vi "_FPGA_Driver_V1.4DIO.vi"(10 "DO":u8) -> (2 "DI":u8)   [LabVIEW 2018]
uses:
  <vilib>/rvi/eio/common/nirviEmuTemplateMethod_errors.vi
  <vilib>/eio/EIONode/EIONode.xnode
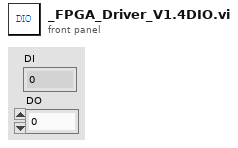
[diagram p1: front panel]
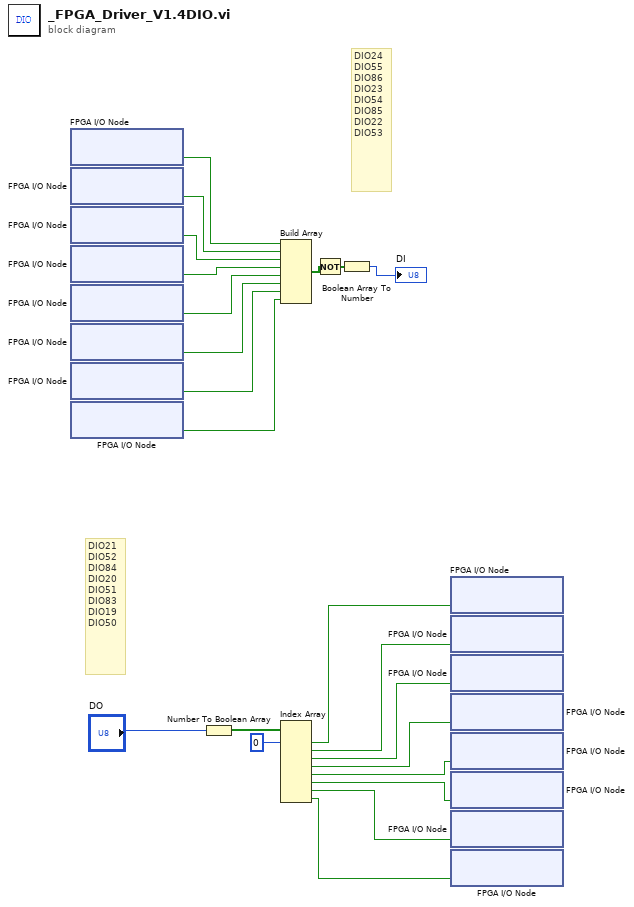
[diagram p0: block diagram]
diagram:
  # "DIO21\nDIO52\nDIO84\nDIO20\nDIO51\nDIO83\nDIO19\nDIO50"
  # "DIO24\nDIO55\nDIO86\nDIO23\nDIO54\nDIO85\nDIO22\nDIO53"
  n1 = xnode "FPGA I/O Node"() -> ("RMC/DIO24"=w22:bool)  [unwired: 1 in, 1 out]
  n2 = xnode "FPGA I/O Node"() -> ("RMC/DIO55"=w21:bool)  [unwired: 1 in, 1 out]
  n3 = xnode "FPGA I/O Node"() -> ("RMC/DIO86"=w20:bool)  [unwired: 1 in, 1 out]
  n4 = xnode "FPGA I/O Node"() -> ("RMC/DIO23"=w19:bool)  [unwired: 1 in, 1 out]
  n5 = xnode "FPGA I/O Node"() -> ("RMC/DIO54"=w18:bool)  [unwired: 1 in, 1 out]
  n6 = xnode "FPGA I/O Node"() -> ("RMC/DIO85"=w17:bool)  [unwired: 1 in, 1 out]
  n7 = xnode "FPGA I/O Node"() -> ("RMC/DIO22"=w16:bool)  [unwired: 1 in, 1 out]
  n8 = xnode "FPGA I/O Node"() -> ("RMC/DIO53"=w15:bool)  [unwired: 1 in, 1 out]
  n9 = Number To Boolean Array(number="DO") -> (Boolean array=w11:bool[])
  n10 = Build Array(w22, w21, w20, w19, w18, w17, w16, w15) -> (w14:bool[])
  n11 = Index Array(array=w11, index #1=0 ("index")) -> (element #1=w9:bool, element #2=w8:bool, element #3=w7:bool, element #4=w6:bool, element #5=w5:bool, element #6=w4:bool, element #7=w3:bool, element #8=w2:bool)  [unwired: 7 in]
  n12 = Not(x=w14) -> (.not. x?=w1:bool[])
  n13 = Boolean Array To Number(Boolean array=w1) -> (number=→"DI":u8)
  n14 = xnode "FPGA I/O Node"("RMC/DIO21"=w9) -> ()  [unwired: 1 in, 1 out]
  n15 = xnode "FPGA I/O Node"("RMC/DIO52"=w8) -> ()  [unwired: 1 in, 1 out]
  n16 = xnode "FPGA I/O Node"("RMC/DIO84"=w7) -> ()  [unwired: 1 in, 1 out]
  n17 = xnode "FPGA I/O Node"("RMC/DIO20"=w6) -> ()  [unwired: 1 in, 1 out]
  n18 = xnode "FPGA I/O Node"("RMC/DIO51"=w5) -> ()  [unwired: 1 in, 1 out]
  n19 = xnode "FPGA I/O Node"("RMC/DIO83"=w4) -> ()  [unwired: 1 in, 1 out]
  n20 = xnode "FPGA I/O Node"("RMC/DIO19"=w3) -> ()  [unwired: 1 in, 1 out]
  n21 = xnode "FPGA I/O Node"("RMC/DIO50"=w2) -> ()  [unwired: 1 in, 1 out]
